vi "Get-file-extension.vi"(8 "error in (no error)":errorcluster, 11 "SettingsFile in":refnum<class "SettingsFile.lvclass">) -> (0 "error out":errorcluster, 2 "File extension":string, 3 "SettingsFile out":refnum<class "SettingsFile.lvclass">)   [LabVIEW 2013, in "SettingsFile.lvlib" / "SettingsFile.lvclass"]
uses:
  SettingsFile.lvclass
  SettingsFile.lvclass/SettingsFile.ctl
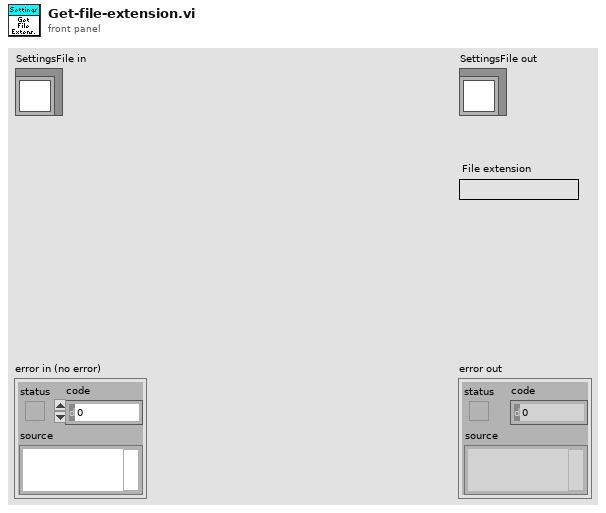
[diagram p1: front panel]
types:
  T1 = enum16{"Not implemented", "Command not recognized", "Invalid input", "No connection", "Timeout", "Invalid file type"}
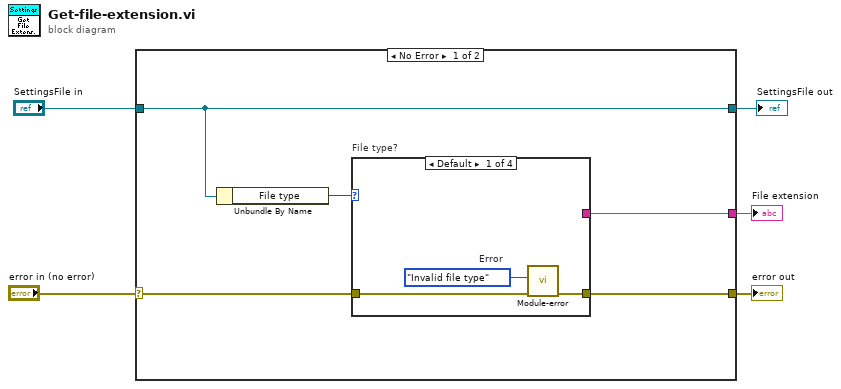
[diagram p0: block diagram]
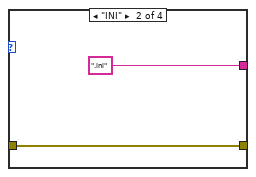
[diagram p2: hidden frame]
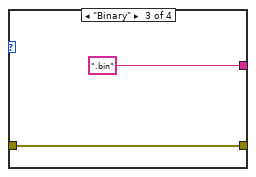
[diagram p3: hidden frame]
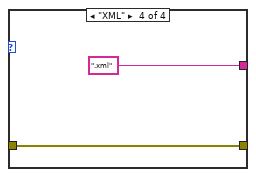
[diagram p4: hidden frame]
diagram:
  n1 = case shown="No Error" "error in (no error)" {
    selector: "error in (no error)" -> [w9 w21]
    tunnel: [w8 w21] -> w4
    tunnel: [w10 w20] -> w2
    tunnel: "SettingsFile in" -> [w10 w20]
    tunnel: [w6 _] -> w1
    frame No Error {
      n2 = Unbundle By Name(w10) -> ("File type"=w7:enum16{"XML", "INI", "Binary"})
      n3 = case "File type?" shown="Default" w7 {
        tunnel: w9 -> [w12 w14 w16 w18]
        tunnel: [w13 w14 w16 w18] -> w8
        tunnel: [_ ".ini" ".bin" ".xml"] -> w6
        frame Default {
          w11 = T1."Invalid file type"  # Error
          n4 = call "Module-error.vi"("error in (no error)"=w12, "Error"=w11) -> ("error out"=w13:errorcluster)  [unwired: 9 in]
        }
        frame "INI" {
        }
        frame "Binary" {
        }
        frame "XML" {
        }
      }
    }
    frame Error {
    }
  }
  "error out" <- w4
  "SettingsFile out" <- w2
  "File extension" <- w1
